vi "detectMSB.vi"(1 "dataInput":dbl) -> (0 "result":bool)   [LabVIEW 2013]
panel:
  out "dataInput 2":dbl
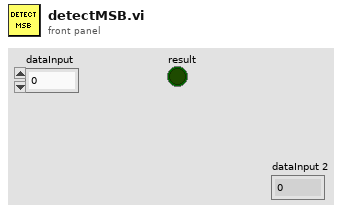
[diagram p1: front panel]
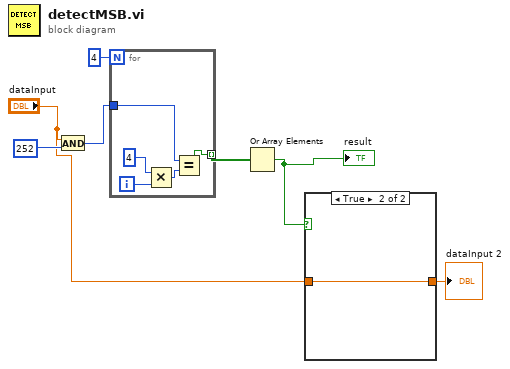
[diagram p0: block diagram]
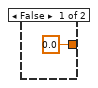
[diagram p2: hidden frame]
diagram:
  n1 = And(x="dataInput", y=u8 252) -> (x .and. y?=w4:i32)
  n2 = for {
    N: 4 -> [_]
    tunnel: w4 -> [w9]
    tunnel: [w8] -> w6 mode=indexing
    i -> [w12]
    n3 = Multiply(x=4, y=w12) -> (x*y=w10:i32)
    n4 = Equal?(x=w9, y=w10) -> (x = y?=w8:bool)
  }
  n5 = Or Array Elements(Boolean array=w6) -> (logical OR=w1:bool)
  "result" <- w1
  n6 = case shown="True" w1 {
    tunnel: "dataInput" -> [_ w14]
    tunnel: [0.0 ("dataInput") w14] -> w2
    frame False {
    }
    frame True {
    }
  }
  "dataInput 2" <- w2
